vi "Get Next Subscriber.vi"(8 "error in (no error)":errorcluster, 10 "Reset":bool, 11 "BroadcastBroker in":refnum<class "BroadcastBroker.lvclass">) -> (0 "error out":errorcluster, 2 "Valid":bool, 3 "BroadcastBroker out":refnum<class "BroadcastBroker.lvclass">)   [LabVIEW 2015, in "BroadcastBroker.lvclass"]
uses:
  BroadcastBroker.lvclass
  BroadcastBroker.lvclass/BroadcastBroker.ctl
panel:
  in  "Topic":string
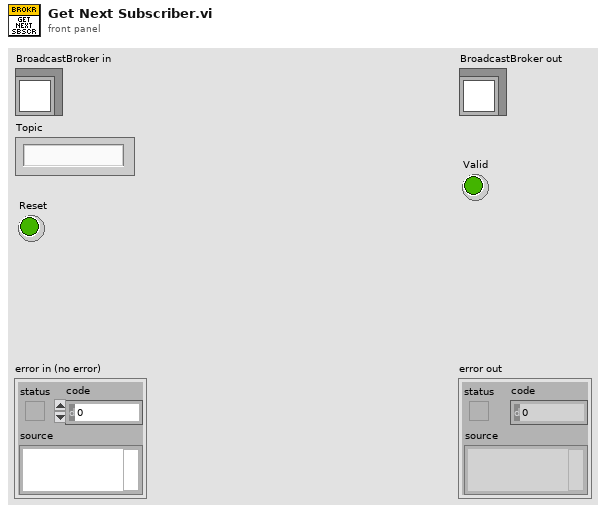
[diagram p1: front panel]
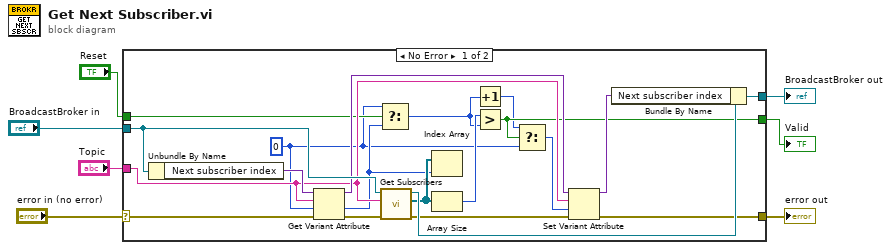
[diagram p0: block diagram]
diagram:
  n1 = case shown="No Error" "error in (no error)" {
    selector: "error in (no error)" -> [w22 w29]
    tunnel: [w14 w29] -> w6
    tunnel: [w17 w28] -> w4
    tunnel: "BroadcastBroker in" -> [w26 w28]
    tunnel: "Topic" -> [w20 _]
    tunnel: "Reset" -> [w19 _]
    tunnel: [w11 _] -> w1
    frame No Error {
      w8 = 0
      n2 = Unbundle By Name(w26) -> ("Next subscriber index"=w25:variant)
      n3 = Get Variant Attribute(Variant=w25, name=w20, default value (empty Variant)=w8, error in=w22) -> (duplicate Variant=w24:variant, value=w18:i32, error out=w21:errorcluster)  [unwired: 1 out]
      n4 = Select(t=w8, s=w19, f=w18) -> (s? t:f=w12:i32)
      n5 = call-dynamic "Get Subscribers.vi"("error in (no error)"=w21, "Topic"=w20, "Broadcaster in"=w26) -> ("error out"=w15:errorcluster, "Subscribers"=w23:refnum<class "Message Enqueuer.lvclass">[], "Broadcaster out"=w27:refnum<class "BroadcastBroker.lvclass">)  [unwired: 5 in, 1 out]
      n6 = Index Array(array=w23, index=w18) -> ()  [unwired: 1 out]
      n7 = Array Size(array=w23) -> (size(s)=w13:i32)
      n8 = Increment(x=w12) -> (x+1=w10:i32)
      n9 = Greater?(x=w13, y=w12) -> (0:w11:bool)
      n10 = Select(t=w10, s=w11, f=w8) -> (s? t:f=w9:i32)
      n11 = Set Variant Attribute(Variant=w24, name=w20, value=w9, error in=w15) -> (Variant out=w16:variant, error out=w14:errorcluster)  [unwired: 1 out]
      n12 = Bundle By Name(cluster=w27, "Next subscriber index"=w16) -> (w17:refnum<class "BroadcastBroker.lvclass">)
    }
    frame Error {
    }
  }
  "error out" <- w6
  "BroadcastBroker out" <- w4
  "Valid" <- w1
